vi "start.vi"(8 "error in (no error)":errorcluster, 9 "spect_depth":u16, 10 "time":dbl, 11 "identifier":string) -> (0 "error out":errorcluster, 3 "function return":u32)   [LabVIEW 2015, in "XGL_DPP.lvlib"]
doc: "EXTERN DECLSPEC unsigned int CALL_CONV start(const char* identifier, const double time);"
uses:
  XGL_DPP.lvlib
  XGL_DPP.dll
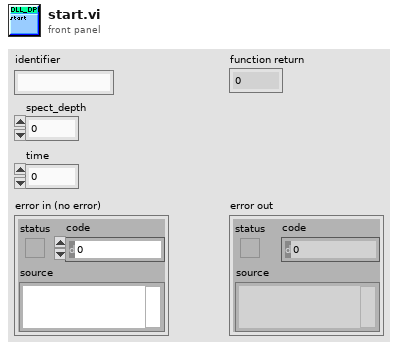
[diagram p1: front panel]
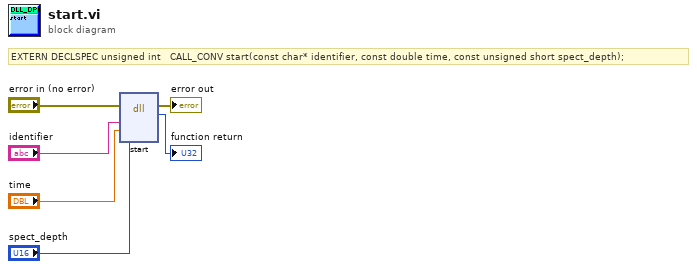
[diagram p0: block diagram]
diagram:
  # "EXTERN DECLSPEC unsigned int   CALL_CONV start(const char* identifier, const double time, const unsigned short spect_depth);"
  n1 = dll-call lib="D:/Users/XRF/Desktop/Dante_acquire4/libs/Dante/XGL_DPP.*" fn="start"(error in="error in (no error)", "identifier"="identifier", "time"="time", "spect_depth"="spect_depth") -> (error out=→"error out":errorcluster, "return type"=→"function return":u32)  [unwired: 5 in, 1 out]
